vi "Handle Last Ack Core.vi"(4 "error in (no error)":errorcluster, 6 "Last Ack":refnum<class "Last Ack.lvclass">, 7 "Cfg Grandmaster in":refnum<class "Cfg Grandmaster.lvclass">) -> (0 "error out":errorcluster, 3 "Cfg Grandmaster out":refnum<class "Cfg Grandmaster.lvclass">)   [LabVIEW 2012, in "Configuration Grandmaster.lvlib" / "Cfg Grandmaster.lvclass"]
doc: "(<B>Filename</B>: Actor Framework.lvlib:Actor.lvclass:Handle Last Ack Core.vi)\n\nDefines how the caller actor responds to the Last Ack message from a nested actor. The Last Ack message is the final message a nested actor sends to its caller before it shuts down. The message contains information about the final state of the nested actor.\n\nBy default, this method does nothing except return any error the nested actor sent. A descendant class may override this method to define behavior."
uses:
  Cfg Grandmaster.lvclass
  <vilib>/ActorFramework/LastAck/Last Ack.lvclass
  <vilib>/ActorFramework/LastAck/Last Ack.lvclass/Last Ack.ctl
  Data Acquisition/Class DAQ Actor/DAQ Actor.lvclass
  Cfg Grandmaster.lvclass/Cfg Grandmaster.ctl
  Actor Nest/Class Actor Nest/Actor Nest.lvclass
  Class FP Ctrls/FP Controls.lvclass
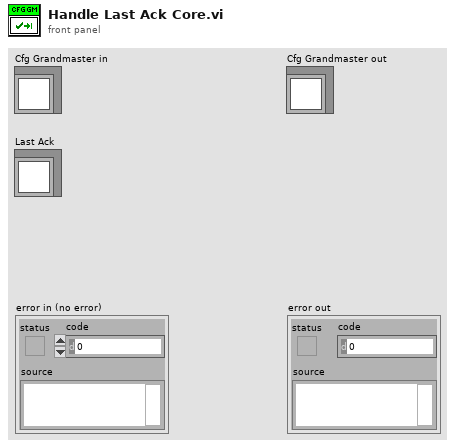
[diagram p1: front panel]
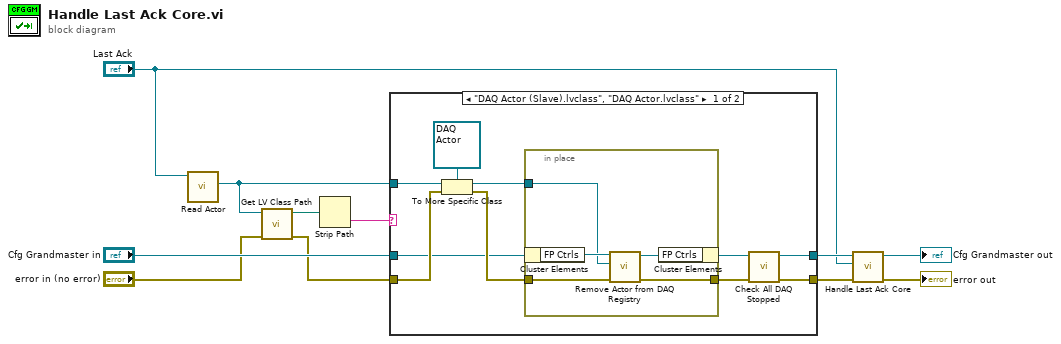
[diagram p0: block diagram]
diagram:
  n1 = call <vilib>:"Read Actor.vi"("Last Ack"="Last Ack") -> ("Actor"=w9:refnum<class "Actor.lvclass">)  [unwired: 10 in]
  n2 = call <vilib>:"Get LV Class Path.vi"("error in (no error)"="error in (no error)", "object"=w9) -> ("error out"=w6:errorcluster, "class path"=w11:path)  [unwired: 8 in]
  n3 = Strip Path(path=w11) -> (name=w10:string)  [unwired: 1 out]
  n4 = case shown="\"DAQ Actor (Slave).lvclass\", \"DAQ Actor.lvclass\"" w10 {
    tunnel: [w13 w27] -> w2
    tunnel: [w14 w28] -> w5
    tunnel: "Cfg Grandmaster in" -> [w17 w28]
    tunnel: w6 -> [w20 w27]
    tunnel: w9 -> [w21 _]
    frame "DAQ Actor (Slave).lvclass", "DAQ Actor.lvclass" {
      n5 = To More Specific Class(target class=refnum<class "DAQ Actor.lvclass"> refnum ("Data Acquisition.lvlib:DAQ Actor.lvclass"), reference=w21, error in=w20) -> (specific class reference=w16:refnum<class "DAQ Actor.lvclass">, error out=w18:errorcluster)
      n6 = in-place {
        in-place-border: [w23] -> w12
        in-place-border: w18 -> [w26]
        in-place-border: w16 -> [w22]
        n7 = in-place-cluster #1(w17) -> ("FP Ctrls"=w25:refnum<class "FP Controls.lvclass">)
        n8 = call "Remove Actor from DAQ Registry.vi"("error in (no error)"=w26, "specific class reference"=w22, "FP Controls in"=w25) -> ("error out"=w23:errorcluster, "FP Controls out"=w24:refnum<class "FP Controls.lvclass">)  [unwired: 7 in]
        n9 = in-place-cluster #1("FP Ctrls"=w24) -> (w15:refnum<class "Cfg Grandmaster.lvclass">)
      }
      n10 = call "Check All DAQ Stopped.vi"("error in (no error)"=w12, "Cfg Grandmaster in"=w15) -> ("error out"=w13:errorcluster, "Cfg Grandmaster out"=w14:refnum<class "Cfg Grandmaster.lvclass">)  [unwired: 8 in]
    }
    frame Default {
    }
  }
  n11 = call-parent "Handle Last Ack Core.vi"("error in (no error)"=w2, "Last Ack"="Last Ack", "Actor Nest in"=w5) -> ("error out"=→"error out":errorcluster, "Actor Nest out"=→"Cfg Grandmaster out":refnum<class "Cfg Grandmaster.lvclass">)  [unwired: 3 in]
